vi "Cleanup.vi"(8 "error in":errorcluster, 11 "Logger Interface in":refnum<class "Logger Interface.lvclass">) -> (0 "error out":errorcluster, 3 "Logger Interface out":refnum<class "Logger Interface.lvclass">)   [LabVIEW 2020, in "Frame Logging.lvlib" / "Logger Interface.lvclass"]
uses:
  Logger Interface.lvclass
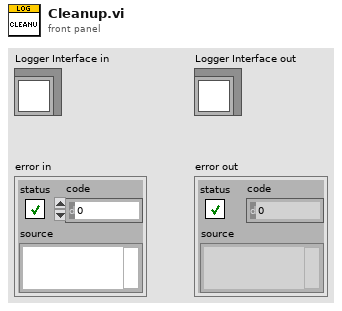
[diagram p1: front panel]
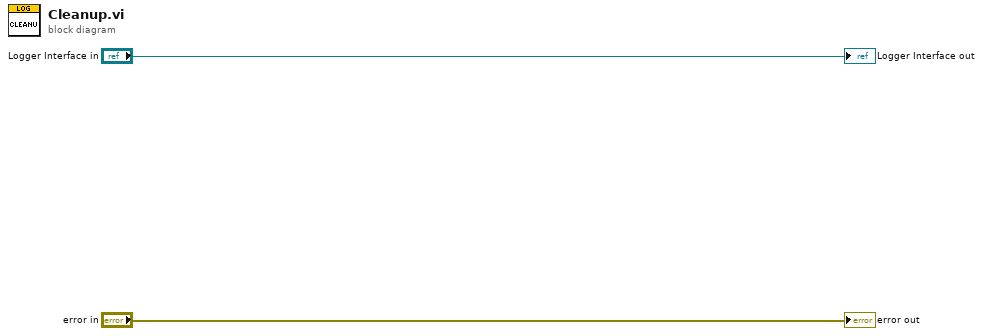
[diagram p0: block diagram]
diagram:
  "error out" <- "error in"
  "Logger Interface out" <- "Logger Interface in"
